vi "Flush Buffer Data.vi"(11 "Buffer Data in":T1) -> (0 "Buffer Empty":bool, 1 "t0":timestamp, 2 "Buffer Data":dbl[][](array[numeric]), 3 "Buffer Data out":T1)   [LabVIEW 2015, in "Triggered Log.lvclass"]
doc: "Flush the data from the buffer and reset the buffer to an empty state. As part of flushing, this VI checks if the data in the circular buffer has wrapped around. If so, it realigns the data in the buffer."
uses:
  Triggered Log.lvclass
  Buffer Data.ctl
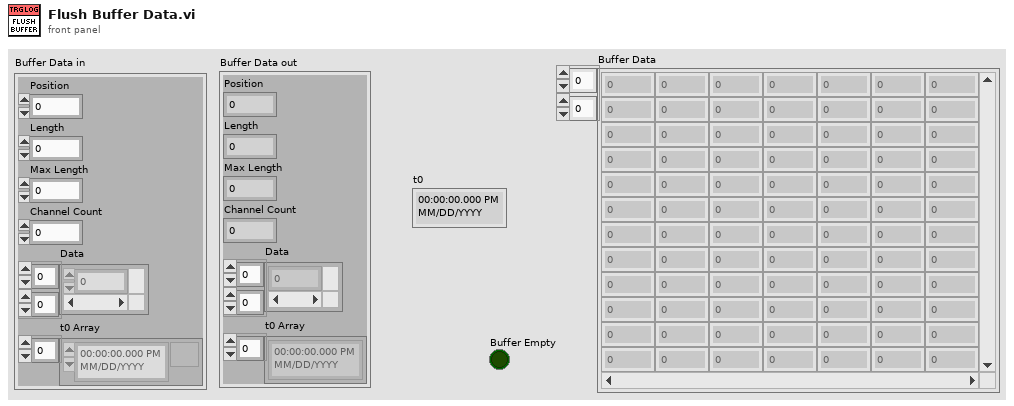
[diagram p1: front panel]
types:
  T1 = typedef "Triggered Log.lvclass/Buffer Data.ctl" = cluster{"Position":i32, "Length":i32, "Max Length":i32, "Channel Count":i32, "Data":dbl[][], "t0 Array":timestamp[]}
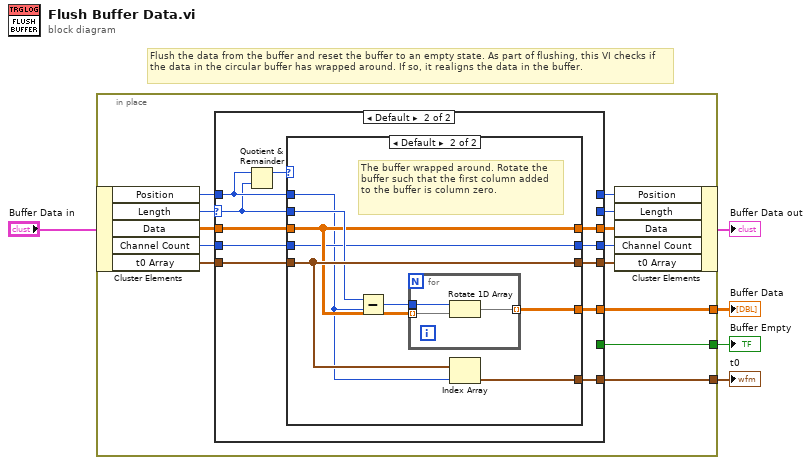
[diagram p0: block diagram]
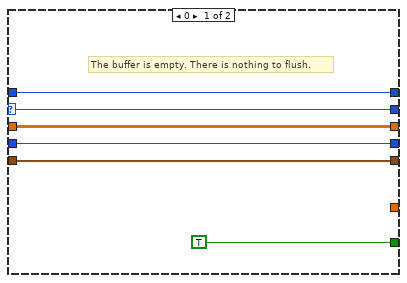
[diagram p2: hidden frame]
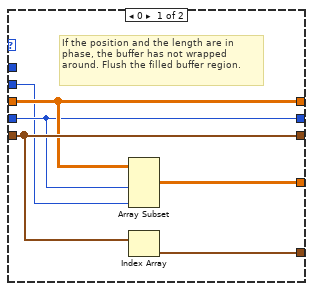
[diagram p3: hidden frame]
diagram:
  # "Flush the data from the buffer and reset the buffer to an empty state. As part of flushing, this VI checks if the data in the circular buffer has wrapped around. If so, it realigns the data in the buffer."
  n1 = in-place {
    in-place-border: [w10] -> w3
    in-place-border: [w9] -> w2
    in-place-border: [w6] -> w1
    n2 = in-place-cluster #1("Buffer Data in") -> ("Position"=w16:i32, "Length"=w11:i32, "Data"=w18:dbl[][], "Channel Count"=w12:i32, "t0 Array"=w7:timestamp[])
    n3 = case shown="Default" w11 {
      selector: w11 -> [w23 w30]
      tunnel: w18 -> [w22 w35]
      tunnel: [w22 w34] -> w17
      tunnel: w16 -> [w24 w33]
      tunnel: [w24 _] -> w15
      tunnel: [w23 _] -> w14
      tunnel: [w21 w32] -> w13
      tunnel: w12 -> [w21 w31]
      tunnel: [_ w29] -> w10
      tunnel: [TRUE _] -> w9
      tunnel: [w19 w27] -> w8
      tunnel: w7 -> [w19 w26]
      tunnel: [_ w25] -> w6
      frame 0 {
        # "The buffer is empty. There is nothing to flush."
      }
      frame Default {
        n4 = Quotient & Remainder(x=w33, y=w30) -> (x-y*floor(x/y)=w28:i32)  [unwired: 1 out]
        n5 = case shown="Default" w28 {
          tunnel: w33 -> [_ w43]
          tunnel: w35 -> [w40 w46]
          tunnel: [w40 w46] -> w34
          tunnel: w30 -> [w38 w47]
          tunnel: [w39 w45] -> w32
          tunnel: w31 -> [w39 w45]
          tunnel: [w37 w48] -> w29
          tunnel: [w41 w49] -> w27
          tunnel: w26 -> [w41 w49]
          tunnel: [w36 w42] -> w25
          frame 0 {
            # "If the position and the length are in phase, the buffer has not wrapped around. Flush the filled buffer region."
            n6 = Array Subset(array=w40, length (row)=w39, length (col)=w38) -> (w37:dbl[][])  [unwired: 2 in]
            n7 = Index Array(array=w41) -> (element=w36:timestamp)  [unwired: 1 in]
          }
          frame Default {
            # "The buffer wrapped around. Rotate the buffer such that the first column added to the buffer is column zero."
            n8 = Subtract(x=w47, y=w43) -> (x-y=w44:i32)
            n9 = for {
              tunnel: [w50] -> w48 mode=indexing
              tunnel: w46 -> [w52] mode=indexing
              tunnel: w44 -> [w51]
              n10 = Rotate 1D Array(1:w52, 2:w51) -> (0:w50:dbl[])
            }
            n11 = Index Array(array=w49, index=w43) -> (element=w42:timestamp)
          }
        }
      }
    }
    n12 = in-place-cluster #1("Position"=w15, "Length"=w14, "Data"=w17, "Channel Count"=w13, "t0 Array"=w8) -> (→"Buffer Data out":T1)
  }
  "Buffer Data" <- w3
  "Buffer Empty" <- w2
  "t0" <- w1
